vi "eval_regex_based.vi"(8 "error in (no error)":errorcluster, 9 "Regex":string[][](array[string]), 10 "Device Type":T1, 11 "SN":string) -> (0 "error out":errorcluster, 1 "Device Type out":T2, 2 "SN ok?":bool, 3 "SN out":string)   [LabVIEW 2024, in "SN Validator.lvlib"]
uses:
  SN Validator.lvlib
  SN_device_type_out.ctl
  SN_device_type.ctl
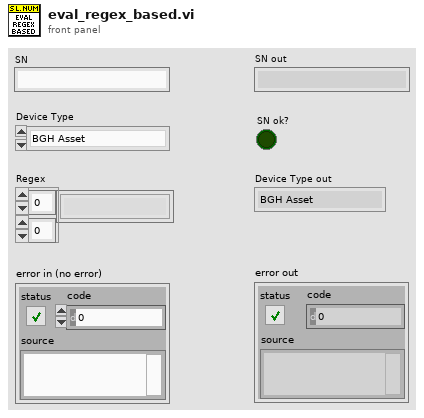
[diagram p1: front panel]
types:
  T1 = typedef "SN Validator.lvlib/SN_device_type.ctl" = enum16{"BGH Asset", "BGH Product", "SAMSUNG Product"}
  T2 = typedef "SN Validator.lvlib/SN_device_type_out.ctl" = enum16{"BGH Asset", "BGH Product", "SAMSUNG Product", "GENERIC Product", "No Product", ""}
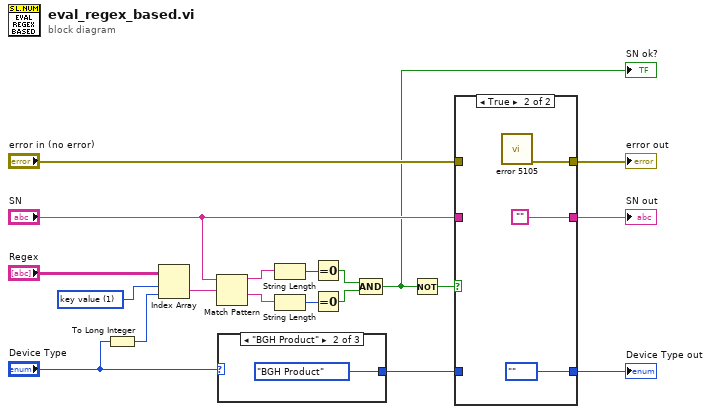
[diagram p0: block diagram]
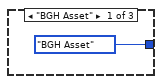
[diagram p3: hidden frame]
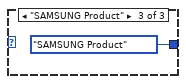
[diagram p4: hidden frame]
diagram:
  w9 = 1 items=["key name", "key value"]
  n1 = To Long Integer(number="Device Type") -> (32bit integer=w13:i32)
  n2 = Index Array(array="Regex", index (row)=w9, index (col)=w13) -> (element=w11:string)
  n3 = Match Pattern(string="SN", regular expression=w11) -> (before substring=w19:string, after substring=w18:string)  [unwired: 1 in, 2 out]
  n4 = case shown="\"BGH Product\"" "Device Type" {
    tunnel: [SN_device_type_out."BGH Asset" ("Device Type out") SN_device_type_out."BGH Product" ("Device Type out") SN_device_type_out."SAMSUNG Product" ("Device Type out")] -> w3
    frame "BGH Asset" {
    }
    frame "BGH Product" {
    }
    frame "SAMSUNG Product" {
    }
  }
  n5 = String Length(string=w19) -> (length=w17:i32)
  n6 = String Length(string=w18) -> (length=w16:i32)
  n7 = Equal To 0?(x=w17) -> (x = 0?=w14:bool)
  n8 = Equal To 0?(x=w16) -> (x = 0?=w15:bool)
  n9 = Compound Arithmetic op=AND(w14, w15) -> (w1:bool)
  "SN ok?" <- w1
  n10 = Not(x=w1) -> (.not. x?=w8:bool)
  n11 = case shown="True" w8 {
    tunnel: "error in (no error)" -> [w23 _]
    tunnel: [w23 w27] -> w6
    tunnel: "SN" -> [w24 _]
    tunnel: [w24 ""] -> w4
    tunnel: w3 -> [w25 _]
    tunnel: [w25 SN_device_type_out."" ("t")] -> w2
    frame False {
    }
    frame True {
      n12 = call "error 5105.vi"() -> ("error out"=w27:errorcluster)  [unwired: 11 in]
    }
  }
  "Device Type out" <- w2
  "error out" <- w6
  "SN out" <- w4
